vi "Get Freq-RPM Spectral Map (DBL).vi"(7 "dB On (T)":bool=TRUE, 8 "error in (no error)":errorcluster, 9 "Gabor template":dbl[](array[numeric]) format="%.2f", 10 "sampling frequency [Hz]":dbl=1.0 format="%.2f", 11 "RefNum in":T1) -> (0 "error out":errorcluster, 1 "quantization info":cluster{"offset":dbl, "multiplier":dbl} {"multiplier" format="%.2f"; "offset" format="%.2f"}, 2 "spectral map":dbl[][](array[numeric]) format="%.2f", 3 "RefNum out":T1, 4 "frequency scale":cluster{"offset":dbl, "multiplier":dbl} {"multiplier" format="%.2f"; "offset" format="%.2f"}, 5 "rpm scale":cluster{"offset":dbl, "multiplier":dbl} {"multiplier" format="%.2f"; "offset" format="%.2f"})   [LabVIEW 2017, in "SoundVib_Gabor.lvlib"]
doc: "Generates a frequency-rpm spectral map of the data block referenced by <B>RefNum in</B>. You can use this polymorphic VI to return <B>spectral map</B> as a 2D array of double-precision, floating-point numbers or a 2D array of 8-bit unsigned integers. You must manually select the polymorphic instance to use. Use the DBL instance to obtain more accurate data. Use the U8 instance to reduce memory usage when the VI displays data."
uses:
  <vilib>/addons/Sound and Vibration/Order Analysis/Gabor Order Tracking/SoundVib_Gabor.lvlib
  <vilib>/addons/Sound and Vibration/Order Analysis/Ref Gabor Order Tracking/GT RefNum.ctl
  <resource>/sndvib.dll
panel:
  # "Get Freq-RPM Spectral Map (DBL)"
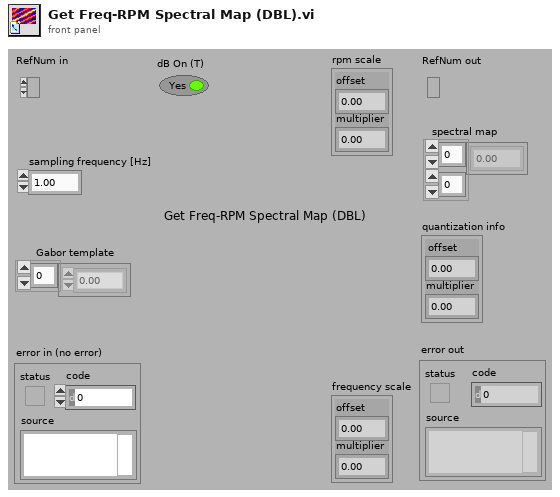
[diagram p1: front panel]
types:
  T1 = typedef "SoundVib_Gabor.lvlib/GT RefNum.ctl" = refnum<k1>
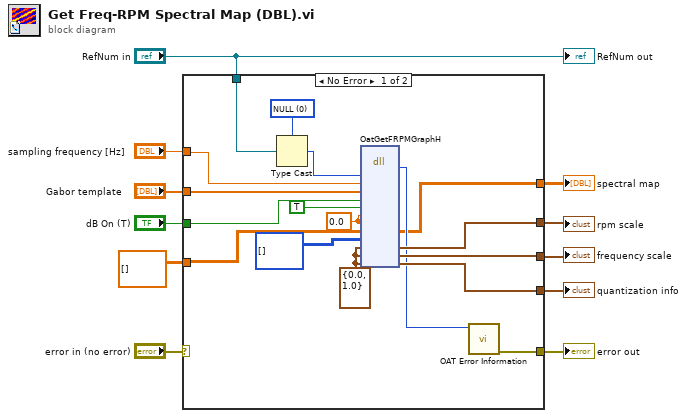
[diagram p0: block diagram]
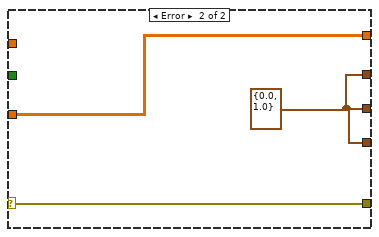
[diagram p2: hidden frame]
diagram:
  n1 = case shown="No Error" "error in (no error)" {
    selector: "error in (no error)" -> [_ w31]
    tunnel: [w28 w31] -> w4
    tunnel: "RefNum in" -> [w26 _]
    tunnel: [w16 w30] -> w11
    tunnel: [w14 w29] -> w8
    tunnel: "Gabor template" -> [w23 _]
    tunnel: "dB On (T)" -> [w22 _]
    tunnel: "sampling frequency [Hz]" -> [w24 _]
    tunnel: [w18 w30] -> w3
    tunnel: [w17 w30] -> w2
    tunnel: dbl[][] [] ("Graph") -> [w12 w29]
    frame No Error {
      w19 = cluster{"offset":dbl, "multiplier":dbl} {"offset"=0.0, "multiplier"=1.0} ("frequency scale")
      w13 = 0.0 ("uCutRatio")
      w27 = u32 0 items=["NULL"]
      n2 = Type Cast(type=w27, x=w26) -> (*(type *) &x=w25:u32)
      n3 = dll-call lib="C:/Program Files (x86)/National Instruments/LabVIEW 2017/resource/sndvib.*" fn="OatGetFRPMGraphH"("Ref In"=w25, "fs"=w24, "CntFreq"=w23, "bLogZ"=w22, "bGetDBL"=TRUE ("dB On (T)"), "uCutRatio"=w13, "dCutRatio"=w13, "DBLGraph"=w12, "U8Graph"=i8[][] [], "XScale"=w19, "YScale"=w19, "ZScale"=w19) -> ("return type"=w15:i32, "DBLGraph"=w14:dbl[][], "XScale"=w18:cluster{"offset":dbl, "multiplier":dbl}, "YScale"=w17:cluster{"offset":dbl, "multiplier":dbl}, "ZScale"=w16:cluster{"offset":dbl, "multiplier":dbl})  [unwired: 11 in, 2 out]
      n4 = call <vilib>:"OAT Error Information.vi"("error code"=w15) -> ("error out"=w28:errorcluster)  [unwired: 6 in]
    }
    frame Error {
      w30 = cluster{"Z Min":dbl, "Z Step":dbl} {"Z Min"=0.0, "Z Step"=1.0}
    }
  }
  "error out" <- w4
  "quantization info" <- w11
  "frequency scale" <- w2
  "rpm scale" <- w3
  "spectral map" <- w8
  "RefNum out" <- "RefNum in"
